vi "Exponential - CM.vi"(1 "Complex Matrix A":T1) -> (0 "e^A":T1)   [LabVIEW 2017, in "NI_Matrix.lvlib"]
doc: "Computes the exponential of the input matrix."
uses:
  <vilib>/Analysis/Matrix/NI_Matrix.lvlib
  <vilib>/Analysis/Matrix/Datatypes/ComplexMatrix.ctl
  <vilib>/Analysis/7linalg.llb/Complex Matrix Exp.vi
  <vilib>/Analysis/NI_AALBase.lvlib
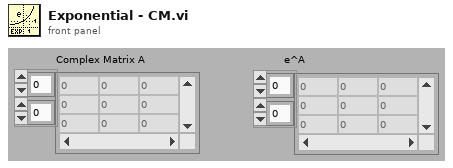
[diagram p1: front panel]
types:
  T1 = typedef "NI_Matrix.lvlib/ComplexMatrix.ctl" = cdb[][]
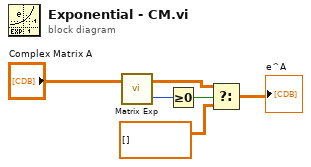
[diagram p0: block diagram]
diagram:
  n1 = call-poly <vilib>:"Matrix Exp.vi"("Input Matrix"="Complex Matrix A") -> ("error"=w3:i32, "Matrix Exp"=w2:T1)  [unwired: 1 in]
  n2 = Greater Or Equal To 0?(x=w3) -> (x >= 0?=w6:bool)
  n3 = Select(t=w2, s=w6, f=T1 [] ("A + B")) -> (s? t:f=→"e^A":T1)
